vi "rwfm_BufferCfgTach.vi"(8 "error in":errorcluster, 9 "Buffer Size [Total Samples]":i32=500000, 11 "Dynamic FPGA VI Reference":refnum<k20>) -> (0 "error out":errorcluster, 1 "Buffer Size [Total Samples]":u32=500000, 3 "FPGA VI Reference Out":refnum<k20>)   [LabVIEW 2017, in "cRIOWfmLib.lvlib"]
doc: "This VI sets the host application's data buffer size, which is critical for maximum data throughput. This buffer is responsible for receiving data coming from the FPGA DMA FIFO. For the continuous case the buffer size should be many times larger than your read size. In the finite case, the timing VIs automatically call this VI and set the buffer size equal to the number of samples in the acquisition."
uses:
  <vilib>/addons/InsightCM/Devices/Shared/Cms/cRIOWfmAcq/cRIOWfmLib.lvlib
  <vilib>/rvi/interface/common/niFpgaWaitOnOcc.vi
  <vilib>/Utility/error.llb/Error Cluster From Error Code.vi
  <vilib>/rvi/interface/nirviMethod/nirviMethod.xnode
  <vilib>/rvi/errors/niLvFpgaMergeErrorWithErrorCode.vi
  <vilib>/FPGAPlugInAG/Dynamic/niLvFpga_ConfigureFifo_Dynamic.vi
  <vilib>/FPGAPlugInAG/Dynamic/niLvFpga_StartFifo_Dynamic.vi
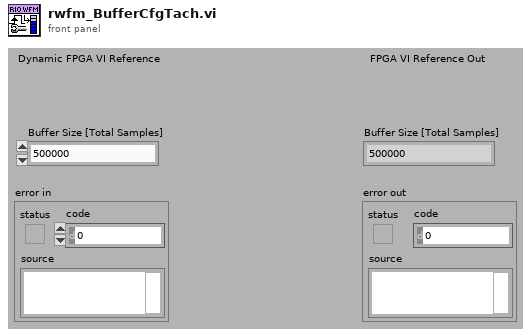
[diagram p1: front panel]
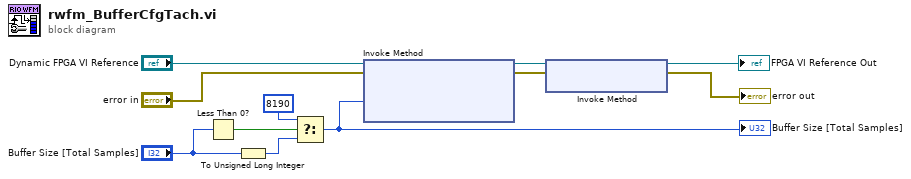
[diagram p0: block diagram]
diagram:
  n1 = Less Than 0?(x="Buffer Size [Total Samples]") -> (x < 0?=w8:bool)
  n2 = To Unsigned Long Integer(number="Buffer Size [Total Samples]") -> (unsigned 32bit integer=w10:u32)
  n3 = Select(t=u32 8190 ("unsigned 32bit integer"), s=w8, f=w10) -> (s? t:f=w2:u32)
  "Buffer Size [Total Samples]" <- w2
  n4 = xnode "Invoke Method"("FPGA VI Reference In"="Dynamic FPGA VI Reference", "error in"="error in", "Requested Depth"=w2) -> ("FPGA VI Reference Out"=w5:refnum<k20>, "error out"=w3:errorcluster)  [unwired: 1 out]
  n5 = xnode "Invoke Method"("FPGA VI Reference In"=w5, "error in"=w3) -> ("FPGA VI Reference Out"=→"FPGA VI Reference Out":refnum<k20>, "error out"=→"error out":errorcluster)
